vi "HB_WriteToLog.vi"(8 "error in (no error)":errorcluster, 10 "Log string":string, 11 "HBDevRef":T1) -> (0 "error out":errorcluster, 3 "HBDevRef":T1)   [LabVIEW 2016]
doc: "Logs the specified string to the currently opened file on the SD card. If no file has been opened, invoking this VI has no effect and the specified string will not be logged. The length of the string must be less than 246 characters or else no data will be logged."
uses:
  <vilib>/Rock Robotics/WPI/SerialPort/WPI_SerialPortRef.ctl
  <vilib>/Utility/error.llb/Error Cluster From Error Code.vi
  <vilib>/ErrorRing/Error Ring.xnode
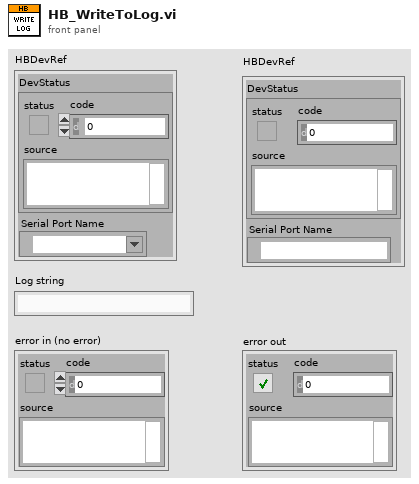
[diagram p1: front panel]
types:
  T1 = typedef "WPI_SerialPortRef.ctl" = cluster{"DevStatus":errorcluster, "Serial Port Name":refnum<visa-resource-name>}
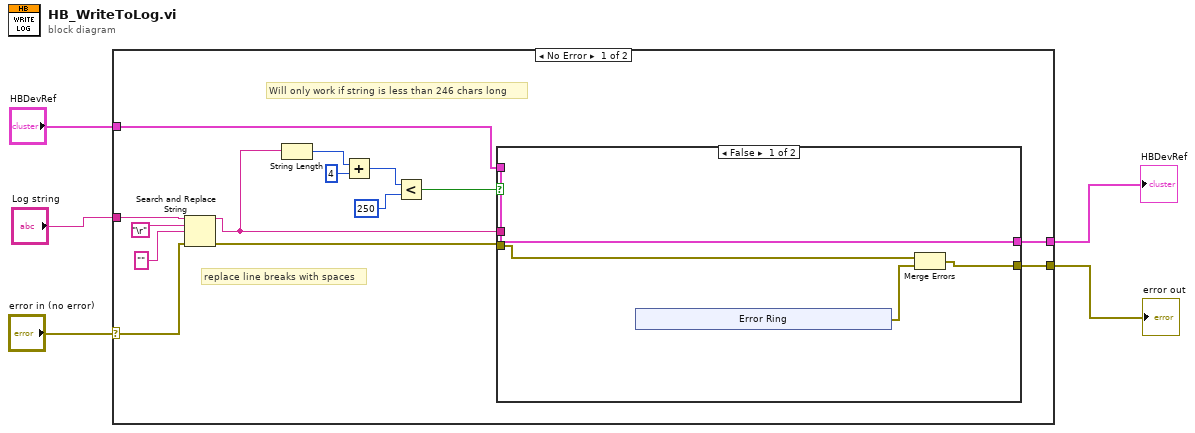
[diagram p0: block diagram]
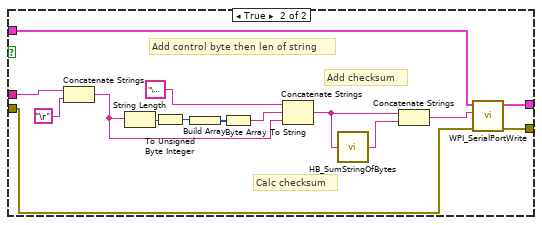
[diagram p2: hidden frame]
diagram:
  n1 = case shown="No Error" "error in (no error)" {
    selector: "error in (no error)" -> [w6 w44]
    tunnel: "Log string" -> [w18 _]
    tunnel: "HBDevRef" -> [w9 w43]
    tunnel: [w8 w43] -> w3
    tunnel: [w7 w44] -> w2
    frame No Error {
      # "Will only work if string is less than 246 chars long"
      # "replace line breaks with spaces"
      n2 = Search and Replace String(input string=w18, search string="\r", replace string="" ("replace string (\"\")"), error in=w6) -> (result string=w12:string, error out=w11:errorcluster)  [unwired: 4 in, 2 out]
      n3 = String Length(string=w12) -> (length=w14:i32)
      n4 = Add(x=w14, y=4) -> (x+y=w16:i32)
      n5 = Less?(x=w16, y=250) -> (x < y?=w13:bool)
      n6 = case shown="False" w13 {
        tunnel: w12 -> [_ w31]
        tunnel: w11 -> [w22 w30]
        tunnel: [w21 w34] -> w8
        tunnel: [w23 w33] -> w7
        tunnel: w9 -> [w21 w32]
        frame False {
          n7 = xnode "Error Ring"() -> ("error out"=w20:errorcluster)
          n8 = Merge Errors(w22, w20) -> (w23:errorcluster)
        }
        frame True {
          # "Add checksum"
          # "Add control byte then len of string"
          # "Calc checksum"
          n9 = Concatenate Strings(w31, "\r") -> (w37:string)
          n10 = String Length(string=w37) -> (length=w39:i32)
          n11 = To Unsigned Byte Integer(number=w39) -> (unsigned 8bit integer=w38:u8)
          n12 = Build Array(w38) -> (w42:u8[])
          n13 = Byte Array To String(unsigned byte array=w42) -> (string=w41:string)
          n14 = Concatenate Strings("\u0001", w41, w37) -> (w28:string)
          n15 = call "HB_SumStringOfBytes.vi"("String Of Bytes"=w28) -> ("Sum as String"=w29:string)
          n16 = Concatenate Strings(w28, w29) -> (w35:string)
          n17 = call <vilib>:"WPI_SerialPortWrite.vi"("error in (no error)"=w30, "Buffer"=w35, "SerialPortRef"=w32) -> ("error out"=w33:errorcluster, "SerialPortRef"=w34:T1)  [unwired: 6 in, 1 out]
        }
      }
    }
    frame Error {
    }
  }
  "HBDevRef" <- w3
  "error out" <- w2
